vi "ResizeFrame.vi"(8 "error in (no error)":errorcluster, 11 "FlatSequenceFrame in":refnum<vi>) -> (0 "error out":errorcluster, 3 "FlatSequenceFrame out":refnum<vi>)   [LabVIEW 2011]
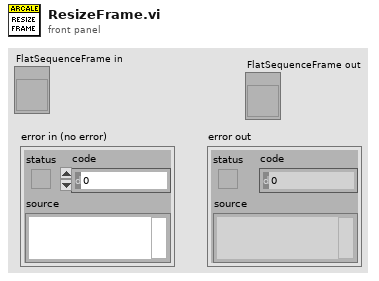
[diagram p1: front panel]
types:
  T1 = typedef "LVRectTypeDef.ctl" = cluster{"left":i16, "top":i16, "right":i16, "bottom":i16}
  T2 = typedef "LVBoundsTypeDef.ctl" = cluster{"Width":u32, "Height":u32}
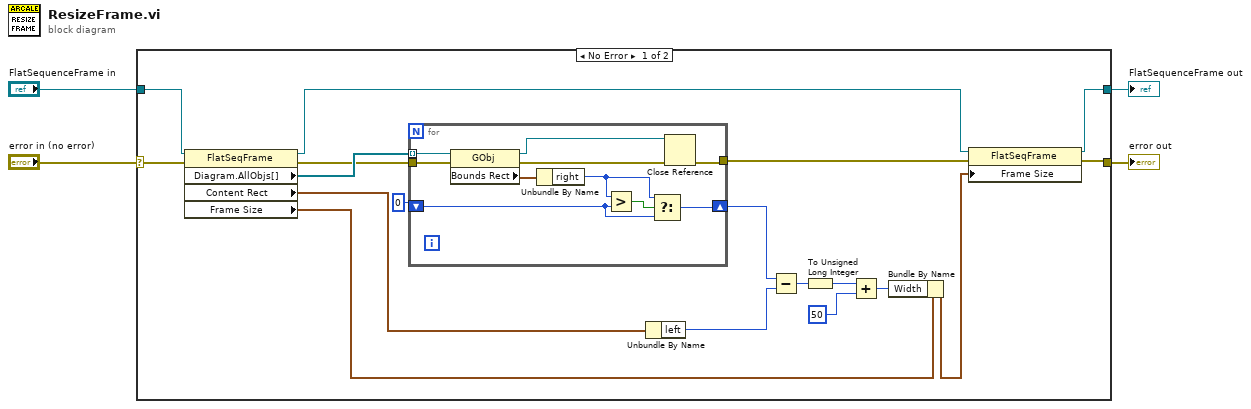
[diagram p0: block diagram]
diagram:
  n1 = case shown="No Error" "error in (no error)" {
    selector: "error in (no error)" -> [w6 w34]
    tunnel: "FlatSequenceFrame in" -> [w22 w33]
    tunnel: [w7 w33] -> w3
    tunnel: [w5 w34] -> w1
    frame No Error {
      n2 = property class="FlatSeqFrame"(reference=w22, error in=w6) -> (reference out=w19:refnum<vi>, error out=w15:errorcluster, "Diagram.AllObjs[]"=w21:refnum<vi>[], "Content Rect"=w20:T1, "Frame Size"=w18:T2)
      n3 = for {
        tunnel: w21 -> [w32] mode=indexing
        shift-right: [w29] -> w13
        shift-left: i16 0 ("right") -> [w27]
        tunnel: w15 -> [w26]
        tunnel: [w24] -> w14
        n4 = property class="GObj"(reference=w32, error in=w26) -> (reference out=w23:refnum<vi>, error out=w25:errorcluster, "Bounds Rect"=w31:T1)
        n5 = Unbundle By Name(w31) -> ("right"=w28:i16)
        n6 = Greater?(x=w28, y=w27) -> (0:w30:bool)
        n7 = Select(t=w28, s=w30, f=w27) -> (s? t:f=w29:i16)
        n8 = Close Reference(reference=w23, error in (no error)=w25) -> (error out=w24:errorcluster)
      }
      n9 = Unbundle By Name(w20) -> ("left"=w12:i16)
      n10 = Subtract(x=w13, y=w12) -> (x-y=w11:i16)
      n11 = To Unsigned Long Integer(number=w11) -> (unsigned 32bit integer=w10:u32)
      n12 = Add(x=w10, y=u32 50) -> (x+y=w8:u32)
      n13 = Bundle By Name(cluster=w18, "Width"=w8) -> (w17:T2)
      n14 = property class="FlatSeqFrame"(reference=w19, error in=w14, "Frame Size"=w17) -> (reference out=w7:refnum<vi>, error out=w5:errorcluster)
    }
    frame Error {
    }
  }
  "FlatSequenceFrame out" <- w3
  "error out" <- w1
